vi "Auto State Machine.vi"   [LabVIEW 2013]
uses:
  typedefs/State Machine/singleUseSubstate.ctl
  typedefs/fg_typedef.ctl
  typedefs/State Machine/subStates.ctl
  typedefs/Vision/vision enable.ctl
  typedefs/DevRef Type.ctl
panel:
  # "A State Machine to Handle One or Two Ball Autonomous"
types:
  T1 = typedef "fg_typedef.ctl" = enum16{"Get", "Set"}
  T2 = typedef "singleUseSubstate.ctl" = enum16{"null", "wait", "shift high", "shift low", "extend shooter", "retract shooter", "latch", "unlatch", "end"}
  T3 = typedef "DevRef Type.ctl" = enum16{"Shooter Solenoid", "Latch Solenoid", "Right Up Sensor", "Right Down Sensor", "Hold Sensor", "2 Ball Switch", "Arm Encoder"}
  T4 = typedef "subStates.ctl" = enum16{"null", "wait", "driver control", "auto", "manual override", "hold position", "rotate", "pickup", "pass", "recover pass", "load", "goto shoot", "shoot high goal", "shoot low goal", "cancel arm", "cancel shooter", "end", "test"}
  T5 = typedef "vision enable.ctl" = enum16{"Enable", "Disable", "Stop"}
  T6 = typedef "WPI_EncoderDevRef.ctl" = cluster{"DevStatus":errorcluster, "EncoderIndex":T7, "CounterIndex":T8, "DistancePerCount":dbl, "Decoding Type":T9}
  T7 = typedef "FPGA_EncoderIdx.ctl" = enum8{"Enc 0", "Enc 1", "Enc 2", "Enc 3", "Invalid"}
  T8 = typedef "FPGA_CounterCtrSystemIndex.ctl" = enum8{"Ctr 0", "Ctr 1", "Ctr 2", "Ctr 3", "Ctr 4", "Ctr 5", "Ctr 6", "Ctr 7", "Invalid"}
  T9 = typedef "WPI_EncoderType.ctl" = enum16{"1x", "2x", "4x"}
  T10 = typedef "WPI_DigitalInputDevRef.ctl" = cluster{"DevStatus":errorcluster, "DIO Channel":T11, "Digital Module":T12}
  T11 = typedef "FPGA_DIOChannel.ctl" = enum8{"DIO 1", "DIO 2", "DIO 3", "DIO 4", "DIO 5", "DIO 6", "DIO 7", "DIO 8", "DIO 9", "DIO 10", "DIO 11", "DIO 12", "DIO 13", "DIO 14", "Invalid"}
  T12 = typedef "FPGA_TypedefDigitalModule.ctl" = enum16{"Digital Module 1", "Digital Module 2"}
  T13 = typedef "vision data.ctl" = cluster{"x":dbl, "y":dbl, "area":dbl, "width":dbl, "height":dbl, "Hot Goal Present?":bool, "distance":dbl}
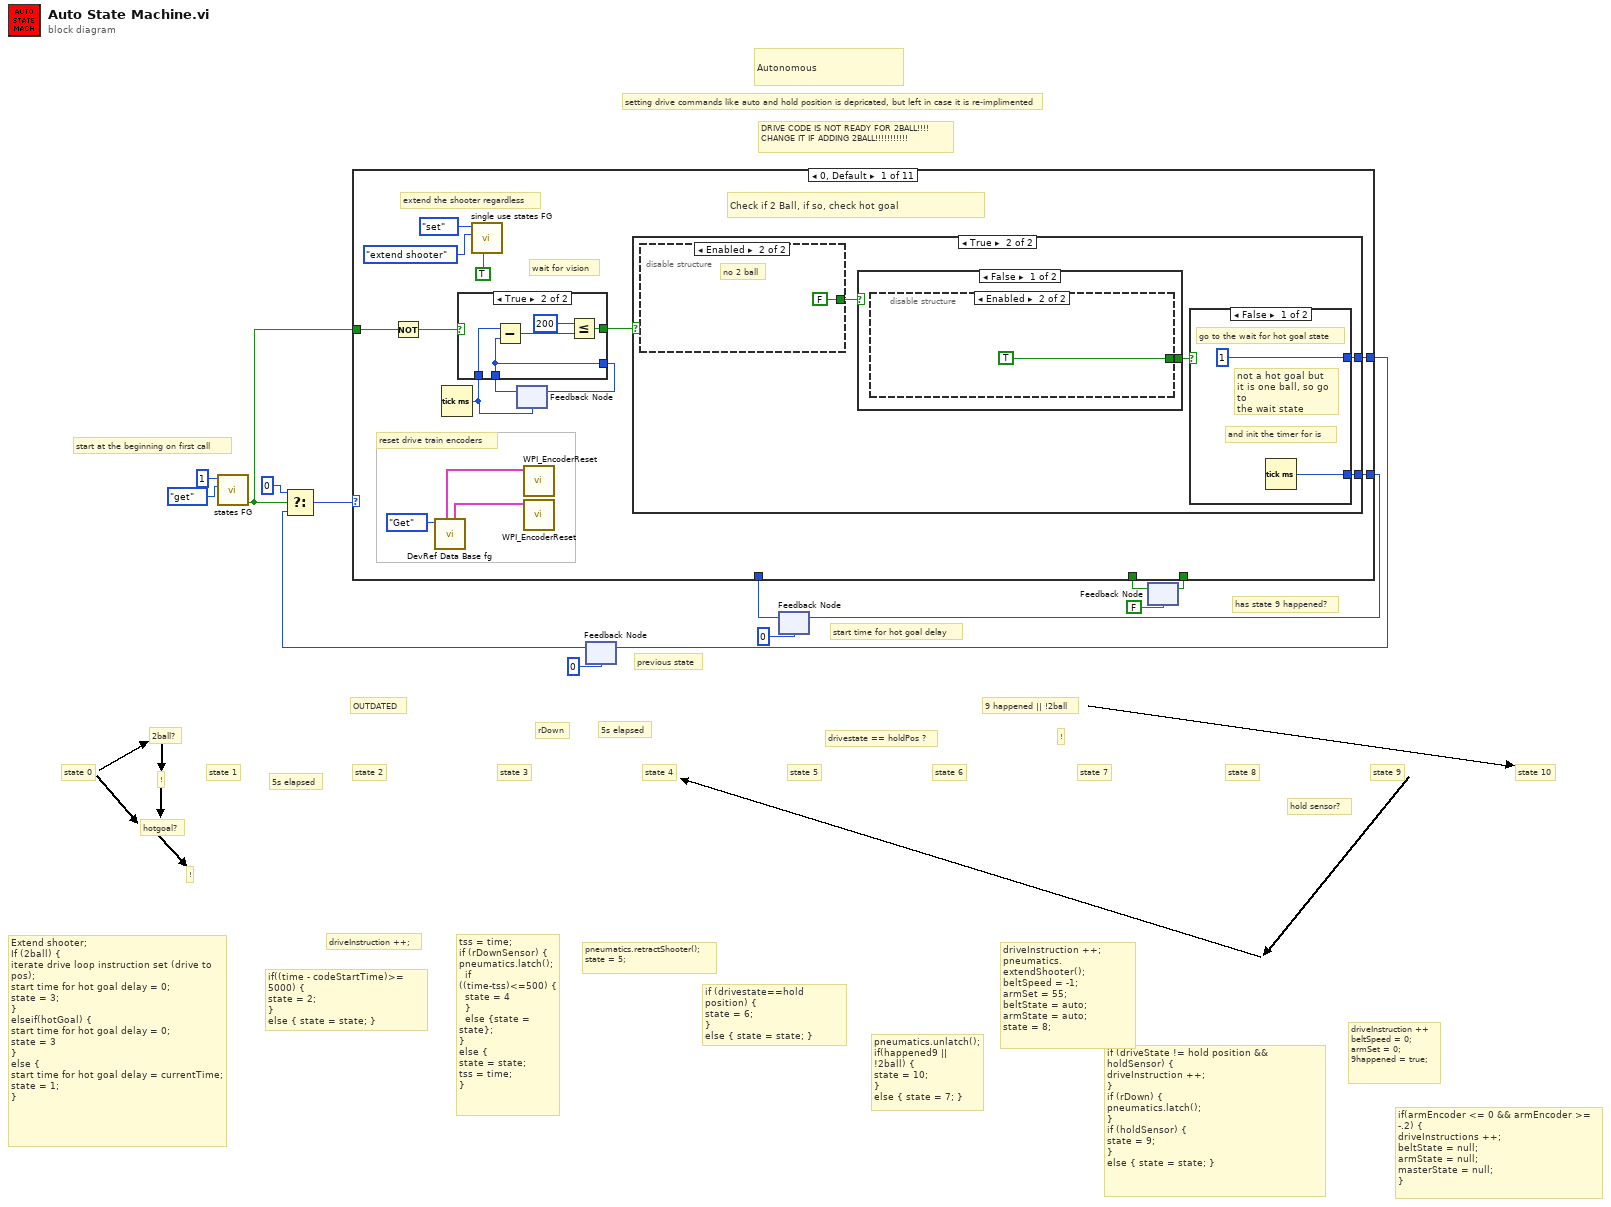
[diagram p0: block diagram]
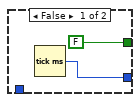
[diagram p2: hidden frame]
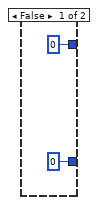
[diagram p3: hidden frame]
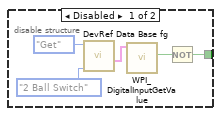
[diagram p4: hidden frame]
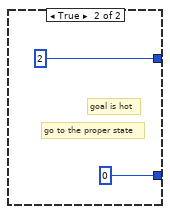
[diagram p5: hidden frame]
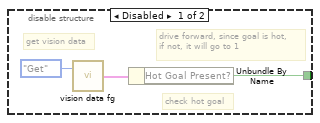
[diagram p6: hidden frame]
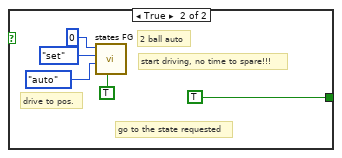
[diagram p7: hidden frame]
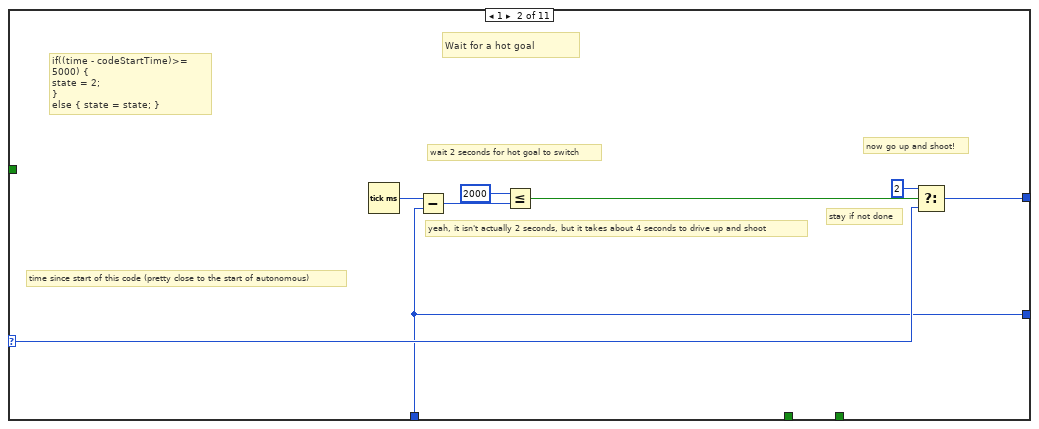
[diagram p8: hidden frame]
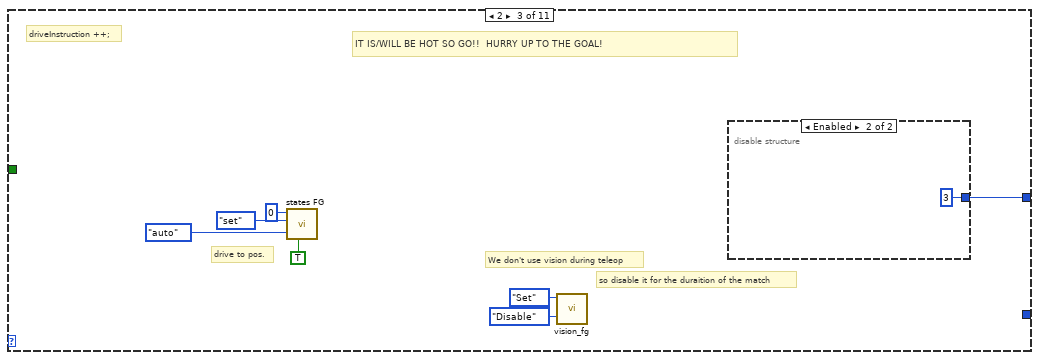
[diagram p9: hidden frame]
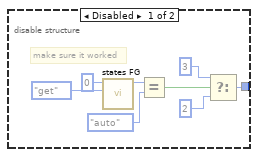
[diagram p10: hidden frame]
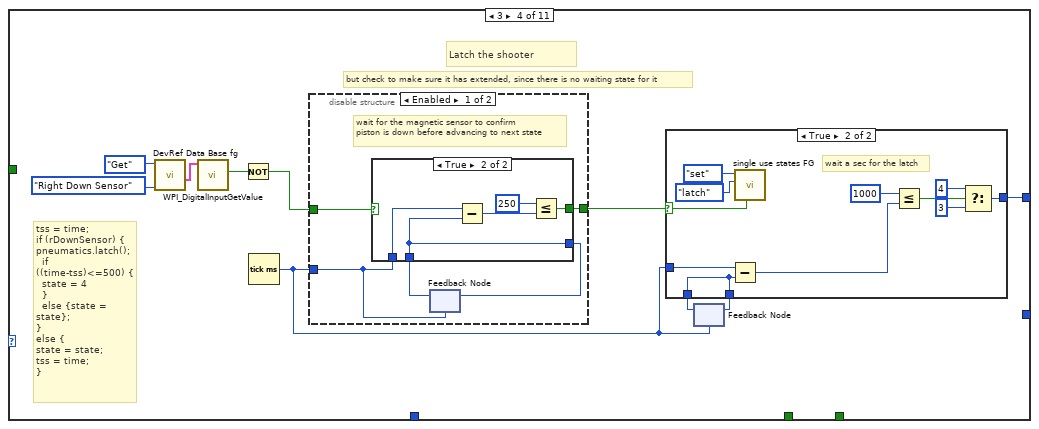
[diagram p11: hidden frame]
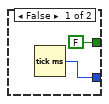
[diagram p12: hidden frame]
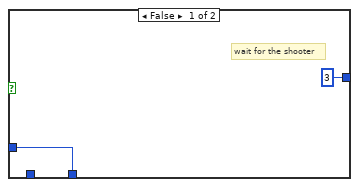
[diagram p14: hidden frame]
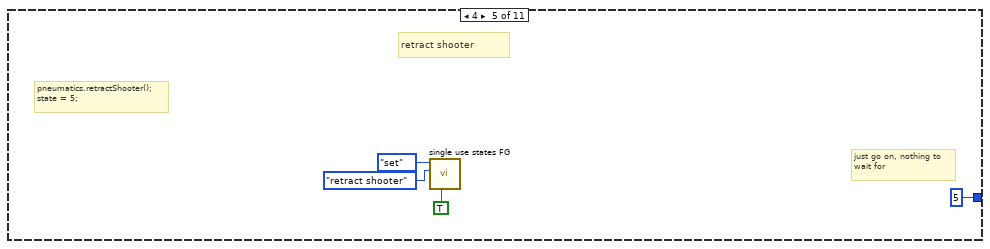
[diagram p15: hidden frame]
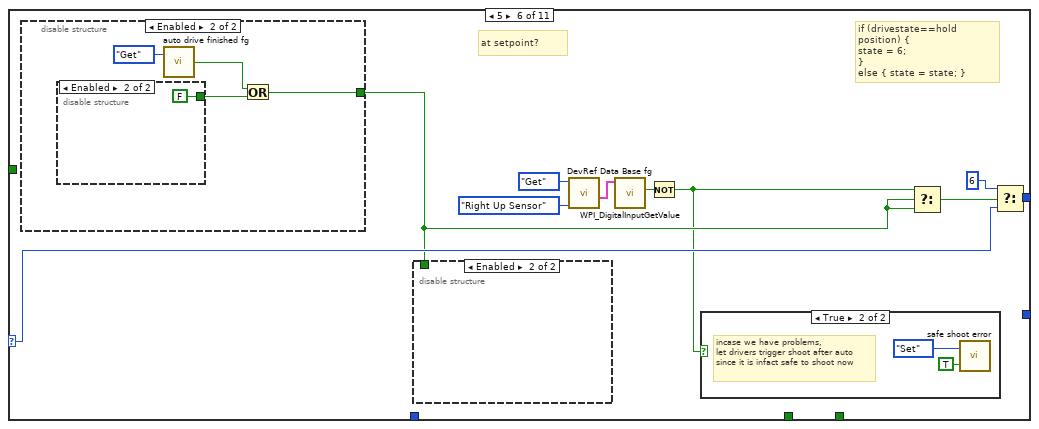
[diagram p16: hidden frame]
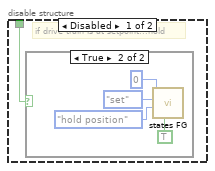
[diagram p17: hidden frame]
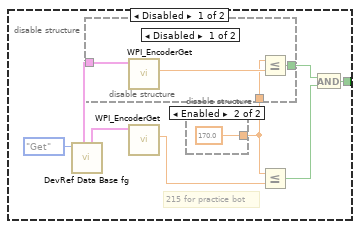
[diagram p19: hidden frame]
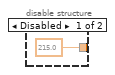
[diagram p20: hidden frame]
diagram:
  # "OUTDATED"
  # "DRIVE CODE IS NOT READY FOR 2BALL!!!!\nCHANGE IT IF ADDING 2BALL!!!!!!!!!!!"
  # "setting drive commands like auto and hold position is depricated, but left in case it is re-implimented"
  # "if(armEncoder <= 0 && armEncoder >= -.2) {\ndriveInstructions ++;\nbeltState = null;\narmState = null;\nmasterState = null;\n}"
  # "driveInstruction ++\nbeltSpeed = 0;\narmSet = 0;\n9happened = true;"
  # "if (driveState != hold position && holdSensor) {\ndriveInstruction ++;\n}\nif (rDown) {\npneumatics.latch();\n}\nif (holdSensor) {\nstate = 9;\n}\nelse { state = state; }"
  # "driveInstruction ++;\npneumatics.extendShooter();\nbeltSpeed = -1;\narmSet = 55;\nbeltState = auto;\narmState = auto;\nstate = 8;"
  # "pneumatics.unlatch();\nif(happened9 || !2ball) {\nstate = 10;\n}\nelse { state = 7; }"
  # "if (drivestate==hold position) {\nstate = 6;\n}\nelse { state = state; }"
  # "pneumatics.retractShooter();\nstate = 5;"
  # "tss = time;\nif (rDownSensor) {\npneumatics.latch();\n  if ((time-tss)<=500) {\n  state = 4\n  }\n  else {state = state};\n}\nelse {\nstate = state;\ntss = time;\n}"
  # "driveInstruction ++;"
  # "if((time - codeStartTime)>= 5000) {\nstate = 2;\n}\nelse { state = state; }"
  # "Extend shooter;\nIf (2ball) {\niterate drive loop instruction set (drive to pos);\nstart time for hot goal delay = 0;\nstate = 3;\n}\nelseif(hotGoal) {\nstart time for hot goal delay = 0;\nstate = 3\n}\nelse {\nstart time for hot goal delay = currentTime;\nstate = 1;\n}"
  # "hold sensor?"
  # "!"
  # "9 happened || !2ball"
  # "drivestate == holdPos ?"
  # "5s elapsed"
  # "rDown"
  # "5s elapsed"
  # "!"
  # "hotgoal?"
  # "!"
  # "state 10"
  # "2ball?"
  # "state 9"
  # "state 8"
  # "state 7"
  # "state 6"
  # "state 5"
  # "state 4"
  # "state 3"
  # "state 2"
  # "state 1"
  # "state 0"
  # "has state 9 happened?"
  # "start time for hot goal delay"
  # "previous state"
  # "start at the beginning on first call"
  # "Autonomous"
  n1 = call "states FG.vi"("menu (get)"=enum16{"set", "get"}."get", "Loop ID"=1) -> ("first call?"=w1:bool)  [unwired: 6 in, 3 out]
  n2 = feedback #1(u8 0) -> (w10:u8)
  n3 = Select(t=u8 0, s=w1, f=w10) -> (s? t:f=w12:u8)
  n4 = feedback #2(u32 0 ("millisecond timer value")) -> (w5:u32)
  n5 = feedback #3(FALSE) -> (w3:bool)
  n6 = case shown="0, Default" w12 {
    selector: w12 -> [_ w63 _ _ _ w135 _ _ w233 _ w269]
    tunnel: [w28 w64 w72 w91 u8 5 ("t") w133 w175 u8 8 ("t") w232 u8 4 ("t") w269] -> w8
    tunnel: [w27 w62 _ _ _ _ _ _ _ _ _] -> w7
    tunnel: w5 -> [_ w62 _ _ _ _ _ _ _ _ _]
    tunnel: [_ _ _ _ _ _ _ _ _ TRUE _] -> w4
    tunnel: w3 -> [_ _ _ _ _ _ w171 _ _ _ _]
    tunnel: w1 -> [w17 _ _ _ _ _ _ _ _ _ _]
    frame 0, Default {
      # "reset drive train encoders"
      # "wait for vision"
      # "extend the shooter regardless"
      # "Check if 2 Ball, if so, check hot goal"
      n7 = Not(x=w17) -> (.not. x?=w16:bool)
      n8 = call "DevRef Data Base fg.vi"("Menu"=fg_typedef."Get") -> ("right drive encoder"=w21:T6, "left drive encoder"=w22:T6)  [unwired: 3 in, 4 out]
      n9 = Tick Count (ms)() -> (millisecond timer value=w20:u32)
      n10 = call "single use states FG.vi"("exit in"=TRUE, "substate"=singleUseSubstate."extend shooter", "menu (get)"=enum16{"set", "get"}."set") -> ()  [unwired: 5 in, 4 out]
      n11 = feedback #4(w20) -> (w18:u32)
      n12 = case shown="True" w16 {
        tunnel: w20 -> [_ w33]
        tunnel: [w30 w31] -> w19
        tunnel: w18 -> [_ w31]
        tunnel: [FALSE w32] -> w15
        frame False {
          n13 = Tick Count (ms)() -> (millisecond timer value=w30:u32)
        }
        frame True {
          n14 = Subtract(x=w33, y=w31) -> (x-y=w35:u32)
          n15 = Less Or Equal?(x=u32 200, y=w35) -> (x <= y?=w32:bool)
        }
      }
      n16 = feedback-in #4(w19) -> ()
      n17 = call <vilib>:"WPI_EncoderReset.vi"("EncoderDevRef"=w22) -> ()  [unwired: 9 in, 2 out]
      n18 = call <vilib>:"WPI_EncoderReset.vi"("EncoderDevRef"=w21) -> ()  [unwired: 9 in, 2 out]
      n19 = case shown="True" w15 {
        tunnel: [u8 0 ("f") w40] -> w28
        tunnel: [u32 0 ("millisecond timer value") w39] -> w27
        frame False {
        }
        frame True {
          n20 = disable-structure shown="Enabled" {
            disable-tunnel: [w44 FALSE] -> w38
            frame Disabled {
              n21 = call "DevRef Data Base fg.vi"("DevRef to Get"=DevRef_Type."2 Ball Switch", "Menu"=fg_typedef."Get") -> ("Selected Sensor"=w46:T10)  [unwired: 2 in, 5 out]
              n22 = call <vilib>:"WPI_DigitalInputGetValue.vi"("DigitalInputDevRef"=w46) -> ("Value"=w45:bool)  [unwired: 8 in, 2 out]
              n23 = Not(x=w45) -> (.not. x?=w44:bool)
            }
            frame Enabled {
              # "no 2 ball"
            }
          }
          n24 = case shown="False" w38 {
            tunnel: [w52 TRUE ("Hot Goal Present?")] -> w41
            frame False {
              n25 = disable-structure shown="Enabled" {
                disable-tunnel: [w53 TRUE ("Hot Goal Present?")] -> w52
                frame Disabled {
                  # "drive forward, since goal is hot,\nif not, it will go to 1"
                  # "check hot goal"
                  # "get vision data"
                  n26 = call "vision data fg.vi"("Menu"=fg_typedef."Get") -> ("Output"=w54:T13)  [unwired: 1 in]
                  n27 = Unbundle By Name(w54) -> ("Hot Goal Present?"=w53:bool)
                }
                frame Enabled {
                }
              }
            }
            frame True {
              # "go to the state requested"
              # "drive to pos."
              # "start driving, no time to spare!!!"
              # "2 ball auto"
              n28 = call "states FG.vi"("exit in"=TRUE, "subState in"=subStates."auto", "menu (get)"=enum16{"set", "get"}."set", "Loop ID"=0) -> ()  [unwired: 4 in, 4 out]
            }
          }
          n29 = case shown="False" w41 {
            tunnel: [u8 1 ("f") u8 2] -> w40
            tunnel: [w49 u32 0 ("millisecond timer value")] -> w39
            frame False {
              # "go to the wait for hot goal state"
              # "and init the timer for is"
              # "not a hot goal but\nit is one ball, so go to\nthe wait state"
              n30 = Tick Count (ms)() -> (millisecond timer value=w49:u32)
            }
            frame True {
              # "go to the proper state"
              # "goal is hot"
            }
          }
        }
      }
    }
    frame 1 {
      # "yeah, it isn't actually 2 seconds, but it takes about 4 seconds to drive up and shoot"
      # "if((time - codeStartTime)>= 5000) {\nstate = 2;\n}\nelse { state = state; }"
      # "now go up and shoot!"
      # "stay if not done"
      # "time since start of this code (pretty close to the start of autonomous)"
      # "wait 2 seconds for hot goal to switch"
      # "Wait for a hot goal"
      n31 = Tick Count (ms)() -> (millisecond timer value=w67:u32)
      n32 = Subtract(x=w67, y=w62) -> (x-y=w69:u32)
      n33 = Less Or Equal?(x=u32 2000, y=w69) -> (x <= y?=w66:bool)
      n34 = Select(t=u8 2, s=w66, f=w63) -> (s? t:f=w64:u8)
    }
    frame 2 {
      # "so disable it for the duraition of the match"
      # "We don't use vision during teleop"
      # "driveInstruction ++;"
      # "drive to pos."
      # "IT IS/WILL BE HOT SO GO!!  HURRY UP TO THE GOAL!"
      n35 = call "states FG.vi"("exit in"=TRUE, "subState in"=subStates."auto", "menu (get)"=enum16{"set", "get"}."set", "Loop ID"=0) -> ()  [unwired: 4 in, 4 out]
      n36 = call "vision_fg.vi"("Action"=vision_enable."Disable", "Menu"=fg_typedef."Set" ("Enum")) -> ()  [unwired: 1 in, 2 out]
      n37 = disable-structure shown="Enabled" {
        disable-tunnel: [w77 u8 3 ("t")] -> w72
        frame Disabled {
          # "make sure it worked"
          n38 = call "states FG.vi"("menu (get)"=enum16{"set", "get"}."get", "Loop ID"=0) -> ("subState out"=w82:T4)  [unwired: 6 in, 3 out]
          n39 = Equal?(x=w82, y=subStates."auto" ("subState in")) -> (x = y?=w80:bool)
          n40 = Select(t=u8 3, s=w80, f=u8 2 ("t")) -> (s? t:f=w77:u8)
        }
        frame Enabled {
        }
      }
    }
    frame 3 {
      # "tss = time;\nif (rDownSensor) {\npneumatics.latch();\n  if ((time-tss)<=500) {\n  state = 4\n  }\n  else {state = state};\n}\nelse {\nstate = state;\ntss = time;\n}"
      # "but check to make sure it has extended, since there is no waiting state for it"
      # "Latch the shooter"
      n41 = call "DevRef Data Base fg.vi"("DevRef to Get"=DevRef_Type."Right Down Sensor", "Menu"=fg_typedef."Get") -> ("Selected Sensor"=w95:T10)  [unwired: 2 in, 5 out]
      n42 = call <vilib>:"WPI_DigitalInputGetValue.vi"("DigitalInputDevRef"=w95) -> ("Value"=w94:bool)  [unwired: 8 in, 2 out]
      n43 = Not(x=w94) -> (.not. x?=w88:bool)
      n44 = Tick Count (ms)() -> (millisecond timer value=w87:u32)
      n45 = disable-structure shown="Enabled" {
        disable-tunnel: w88 -> [w100 w108]
        disable-tunnel: [w97 w108] -> w86
        disable-tunnel: w87 -> [w96 _]
        frame Enabled {
          # "wait for the magnetic sensor to confirm \npiston is down before advancing to next state"
          n46 = feedback #5(w96) -> (w98:u32)
          n47 = case shown="True" w100 {
            tunnel: w96 -> [_ w105]
            tunnel: [w102 w103] -> w99
            tunnel: w98 -> [_ w103]
            tunnel: [FALSE w104] -> w97
            frame False {
              n48 = Tick Count (ms)() -> (millisecond timer value=w102:u32)
            }
            frame True {
              n49 = Subtract(x=w105, y=w103) -> (x-y=w107:u32)
              n50 = Less Or Equal?(x=u32 250, y=w107) -> (x <= y?=w104:bool)
            }
          }
          n51 = feedback-in #5(w99) -> ()
        }
        frame Disabled {
        }
      }
      n52 = feedback #6(w87) -> (w92:u32)
      n53 = case shown="True" w86 {
        selector: w86 -> [_ w117]
        tunnel: [w109 w119] -> w93
        tunnel: w92 -> [_ w119]
        tunnel: w87 -> [w109 w118]
        tunnel: [u8 3 ("f") w112] -> w91
        frame False {
          # "wait for the shooter"
        }
        frame True {
          # "wait a sec for the latch"
          n54 = Subtract(x=w118, y=w119) -> (x-y=w114:u32)
          n55 = call "single use states FG.vi"("exit in"=w117, "substate"=singleUseSubstate."latch", "menu (get)"=enum16{"set", "get"}."set") -> ()  [unwired: 5 in, 4 out]
          n56 = Less Or Equal?(x=u32 1000, y=w114) -> (x <= y?=w111:bool)
          n57 = Select(t=u8 4, s=w111, f=u8 3) -> (s? t:f=w112:u8)
        }
      }
      n58 = feedback-in #6(w93) -> ()
    }
    frame 4 {
      # "pneumatics.retractShooter();\nstate = 5;"
      # "just go on, nothing to\nwait for"
      # "retract shooter"
      n59 = call "single use states FG.vi"("exit in"=TRUE, "substate"=singleUseSubstate."retract shooter", "menu (get)"=enum16{"set", "get"}."set") -> ()  [unwired: 5 in, 4 out]
    }
    frame 5 {
      # "if (drivestate==hold position) {\nstate = 6;\n}\nelse { state = state; }"
      # "at setpoint?"
      n60 = disable-structure shown="Enabled" {
        disable-tunnel: [w141 w156] -> w127
        frame Disabled {
          # "215 for practice bot"
          n61 = call "DevRef Data Base fg.vi"("Menu"=fg_typedef."Get") -> ("right drive encoder"=w147:T6, "left drive encoder"=w146:T6)  [unwired: 3 in, 4 out]
          n62 = call <vilib>:"WPI_EncoderGet.vi"("EncoderDevRef"=w147) -> ("Distance"=w145:dbl)  [unwired: 5 in, 5 out]
          n63 = disable-structure shown="Enabled" {
            disable-tunnel: [215.0 ("x") 170.0 ("x")] -> w142
            frame Disabled {
            }
            frame Enabled {
            }
          }
          n64 = disable-structure shown="Disabled" {
            disable-tunnel: w146 -> [w154 _]
            disable-tunnel: [w152 TRUE] -> w144
            disable-tunnel: w142 -> [w151 _]
            frame Disabled {
              n65 = call <vilib>:"WPI_EncoderGet.vi"("EncoderDevRef"=w154) -> ("Distance"=w153:dbl)  [unwired: 5 in, 5 out]
              n66 = Less Or Equal?(x=w151, y=w153) -> (x <= y?=w152:bool)
            }
            frame Enabled {
            }
          }
          n67 = Less Or Equal?(x=w142, y=w145) -> (x <= y?=w143:bool)
          n68 = And(x=w144, y=w143) -> (x .and. y?=w141:bool)
        }
        frame Enabled {
          n69 = disable-structure shown="Enabled" {
            disable-tunnel: [w160 FALSE] -> w157
            frame Disabled {
              # "check if drive is in hold"
              n70 = call "states FG.vi"("menu (get)"=enum16{"set", "get"}."get", "Loop ID"=0) -> ("subState out"=w162:T4)  [unwired: 6 in, 3 out]
              n71 = Equal?(x=w162, y=subStates."hold position" ("subState in")) -> (x = y?=w160:bool)
            }
            frame Enabled {
            }
          }
          n72 = call "auto drive finished fg.vi"("Menu"=fg_typedef."Get") -> ("Done"=w158:bool)  [unwired: 1 in]
          n73 = Or(x=w158, y=w157) -> (x .or. y?=w156:bool)
        }
      }
      n74 = disable-structure shown="Enabled" {
        disable-tunnel: w127 -> [w136 _]
        frame Disabled {
          # "if drive train is at setpoint...hold"
          n75 = case shown="True" w136 {
            frame False {
            }
            frame True {
              n76 = call "states FG.vi"("exit in"=TRUE, "subState in"=subStates."hold position" ("y"), "menu (get)"=enum16{"set", "get"}."set", "Loop ID"=0) -> ()  [unwired: 4 in, 4 out]
            }
          }
        }
        frame Enabled {
        }
      }
      n77 = call "DevRef Data Base fg.vi"("DevRef to Get"=DevRef_Type."Right Up Sensor", "Menu"=fg_typedef."Get") -> ("Selected Sensor"=w132:T10)  [unwired: 2 in, 5 out]
      n78 = call <vilib>:"WPI_DigitalInputGetValue.vi"("DigitalInputDevRef"=w132) -> ("Value"=w131:bool)  [unwired: 8 in, 2 out]
      n79 = Not(x=w131) -> (.not. x?=w126:bool)
      n80 = case shown="True" w126 {
        frame False {
        }
        frame True {
          # "incase we have problems,\nlet drivers trigger shoot after auto\nsince it is infact safe to shoot now"
          n81 = call "safe shoot error.vi"("Can Shoot Safely?"=TRUE, "Menu"=fg_typedef."Set") -> ()  [unwired: 1 out]
        }
      }
      n82 = Select(t=w126, s=w127, f=w127) -> (s? t:f=w128:bool)
      n83 = Select(t=u8 6, s=w128, f=w135) -> (s? t:f=w133:u8)
    }
    frame 6 {
      w169 = FALSE ("Can Shoot Safely?")
      w168 = fg_typedef."Set" ("Menu")
      # "no 2 ball auto ever (as of now)"
      # "unlatch shooter"
      # "SHOOT!!!"
      n84 = call "safe shoot error.vi"("Can Shoot Safely?"=w169, "Menu"=w168) -> ()  [unwired: 1 out]
      n85 = call "auto drive finished fg.vi"("Done?"=w169, "Menu"=w168) -> ()  [unwired: 1 out]
      n86 = call "single use states FG.vi"("exit in"=TRUE, "substate"=singleUseSubstate."unlatch", "menu (get)"=enum16{"set", "get"}."set") -> ()  [unwired: 5 in, 4 out]
      n87 = disable-structure shown="Enabled" {
        disable-tunnel: [w178 TRUE ("Value")] -> w170
        frame Disabled {
          n88 = call "DevRef Data Base fg.vi"("DevRef to Get"=DevRef_Type."2 Ball Switch", "Menu"=fg_typedef."Get") -> ("Selected Sensor"=w179:T10)  [unwired: 2 in, 5 out]
          n89 = call <vilib>:"WPI_DigitalInputGetValue.vi"("DigitalInputDevRef"=w179) -> ("Value"=w178:bool)  [unwired: 8 in, 2 out]
        }
        frame Enabled {
        }
      }
      n90 = disable-structure shown="Enabled" {
        disable-tunnel: [w187 w190] -> w175
        disable-tunnel: w171 -> [w185 w194]
        disable-tunnel: w170 -> [w184 w189]
        frame Disabled {
          # "pneumatics.unlatch();\nif(happened9) {\nstate = 10;\n}\nelseif(2ball) {\nstate = 7\n}\nelse {\nstate = 10\n}"
          # "if 2 ball was done,\ngo on to 7"
          # "prepare for a 2nd ball"
          # "null if done"
          n91 = Not(x=w184) -> (.not. x?=w181:bool)
          n92 = Select(t=FALSE, s=w185, f=w181) -> (s? t:f=w182:bool)
          n93 = Select(t=u8 7, s=w182, f=u8 10 ("t")) -> (s? t:f=w187:u8)
        }
        frame Enabled {
          # "pneumatics.unlatch();\nif(happened9 || !2ball) {\nstate = 10;\n}\nelse { state = 7; }"
          n94 = disable-structure shown="Enabled" {
            disable-tunnel: w194 -> [w197 _]
            disable-tunnel: [w196 w198] -> w193
            disable-tunnel: w189 -> [w195 w198]
            frame Disabled {
              n95 = Or(x=w195, y=w197) -> (x .or. y?=w196:bool)
            }
            frame Enabled {
            }
          }
          n96 = Select(t=u8 10, s=w193, f=u8 7 ("t")) -> (s? t:f=w190:u8)
        }
      }
    }
    frame 7 {
      # "drive back now"
      # "prepare for a ball"
      # "arm to up position"
      # "enable belts and arm"
      # "driveInstruction ++;\npneumatics.extendShooter();\nbeltSpeed = -1;\narmSet = 55;\nbeltState = auto;\narmState = auto;\nstate = 8;"
      # "belts in"
      # "run load commands, drive backwards"
      n97 = call "states FG.vi"("exit in"=TRUE, "menu (get)"=enum16{"set", "get"}."set", "Loop ID"=0) -> ()  [unwired: 5 in, 4 out]
      n98 = call "single use states FG.vi"("exit in"=TRUE, "substate"=singleUseSubstate."extend shooter", "menu (get)"=enum16{"set", "get"}."set") -> ()  [unwired: 5 in, 4 out]
      n99 = call "Arm Setpoint FG.vi"("Setpoint In"=55.0, "Menu"=fg_typedef."Set") -> ()  [unwired: 1 out]
      n100 = call "Belt Speed FG.vi"("Speed In"=-1.0, "Menu"=fg_typedef."Set") -> ()  [unwired: 1 out]
      n101 = call "states FG.vi"("exit in"=TRUE, "subState in"=subStates."auto", "menu (get)"=enum16{"set", "get"}."set", "Loop ID"=2) -> ()  [unwired: 4 in, 4 out]
      n102 = call "states FG.vi"("exit in"=TRUE, "subState in"=subStates."auto", "menu (get)"=enum16{"set", "get"}."set", "Loop ID"=3) -> ()  [unwired: 4 in, 4 out]
    }
    frame 8 {
      # "if (driveState != hold position && holdSensor) {\ndriveInstruction ++;\n}\nif (rDown) {\npneumatics.latch();\n}\nif (holdSensor) {\nstate = 9;\n}\nelse { state = state; }"
      # "latch if extended"
      # "have ball?"
      n103 = disable-structure shown="Enabled" {
        disable-tunnel: [w235 w240] -> w227
        frame Disabled {
          n104 = call "states FG.vi"("menu (get)"=enum16{"set", "get"}."get", "Loop ID"=0) -> ("subState out"=w237:T4)  [unwired: 6 in, 3 out]
          n105 = Not Equal?(x=w237, y=subStates."hold position") -> (x != y?=w235:bool)
        }
        frame Enabled {
          # "if it is close enough..."
          n106 = call "DevRef Data Base fg.vi"("Menu"=fg_typedef."Get") -> ("right drive encoder"=w242:T6, "left drive encoder"=w241:T6)  [unwired: 3 in, 4 out]
          n107 = call <vilib>:"WPI_EncoderGet.vi"("EncoderDevRef"=w241) -> ("Distance"=w249:dbl)  [unwired: 5 in, 5 out]
          n108 = call <vilib>:"WPI_EncoderGet.vi"("EncoderDevRef"=w242) -> ("Distance"=w248:dbl)  [unwired: 5 in, 5 out]
          n109 = Add(x=w249, y=w248) -> (x+y=w247:dbl)
          n110 = Divide(x=w247, y=2.0) -> (x/y=w245:dbl)
          n111 = Greater Or Equal?(x=10.0, y=w245) -> (x >= y?=w240:bool)
        }
      }
      n112 = call "DevRef Data Base fg.vi"("DevRef to Get"=DevRef_Type."Hold Sensor", "Menu"=fg_typedef."Get") -> ("Selected Sensor"=w231:T10)  [unwired: 2 in, 5 out]
      n113 = call "DevRef Data Base fg.vi"("DevRef to Get"=DevRef_Type."Right Down Sensor", "Menu"=fg_typedef."Get") -> ("Selected Sensor"=w226:T10)  [unwired: 2 in, 5 out]
      n114 = call <vilib>:"WPI_DigitalInputGetValue.vi"("DigitalInputDevRef"=w231) -> ("Value"=w230:bool)  [unwired: 8 in, 2 out]
      n115 = call <vilib>:"WPI_DigitalInputGetValue.vi"("DigitalInputDevRef"=w226) -> ("Value"=w225:bool)  [unwired: 8 in, 2 out]
      n116 = Not(x=w225) -> (.not. x?=w224:bool)
      n117 = Not(x=w230) -> (.not. x?=w228:bool)
      n118 = case shown="True" w224 {
        tunnel: [FALSE w251] -> w222
        frame False {
          # "wait.."
        }
        frame True {
          w251 = TRUE
          n119 = call "single use states FG.vi"("exit in"=w251, "substate"=singleUseSubstate."latch", "menu (get)"=enum16{"set", "get"}."set") -> ()  [unwired: 5 in, 4 out]
        }
      }
      n120 = And(x=w227, y=w228) -> (x .and. y?=w229:bool)
      n121 = case shown="True" w229 {
        frame False {
        }
        frame True {
          # "stop drive if it is not already"
          n122 = call "states FG.vi"("exit in"=TRUE, "subState in"=subStates."hold position", "menu (get)"=enum16{"set", "get"}."set", "Loop ID"=0) -> ()  [unwired: 4 in, 4 out]
        }
      }
      n123 = And(x=w228, y=w222) -> (x .and. y?=w223:bool)
      n124 = Select(t=u8 9, s=w223, f=w233) -> (s? t:f=w232:u8)
    }
    frame 9 {
      # "driveInstruction ++\nbeltSpeed = 0;\narmSet = 0;\n9happened = true;"
      # "arm down"
      # "belts off"
      # "sends drive into auto state (due to autonomous code setup)"
      # "drive to pos."
      # "drive forward, arm down, belts off"
      n125 = call "states FG.vi"("exit in"=TRUE, "subState in"=subStates."auto", "menu (get)"=enum16{"set", "get"}."set", "Loop ID"=0) -> ()  [unwired: 4 in, 4 out]
      n126 = call "Arm Setpoint FG.vi"("Setpoint In"=0.0, "Menu"=fg_typedef."Set") -> ()  [unwired: 1 out]
      n127 = call "Belt Speed FG.vi"("Speed In"=0.0, "Menu"=fg_typedef."Set") -> ()  [unwired: 1 out]
    }
    frame 10 {
      # "if(armEncoder <= 0 && armEncoder >= -.2) {\ndriveInstructions ++;\nbeltState = null;\narmState = null;\nmasterState = null;\n}"
      # "null all the things"
      n128 = disable-structure shown="Enabled" {
        disable-tunnel: [w272 TRUE] -> w268
        frame Disabled {
          n129 = call "DevRef Data Base fg.vi"("DevRef to Get"=DevRef_Type."2 Ball Switch", "Menu"=fg_typedef."Get") -> ("Selected Encoder"=w276:T6)  [unwired: 2 in, 5 out]
          n130 = call <vilib>:"WPI_EncoderGet.vi"("EncoderDevRef"=w276) -> ("Distance"=w275:dbl)  [unwired: 5 in, 5 out]
          n131 = In Range and Coerce(upper limit=1.0, x=w275, lower limit=-0.4) -> (In Range?=w272:bool)  [unwired: 1 out]
        }
        frame Enabled {
        }
      }
      n132 = case shown="True" w268 {
        frame False {
        }
        frame True {
          # "null things"
          n133 = call "states FG.vi"("exit in"=TRUE, "subState in"=subStates."null", "menu (get)"=enum16{"set", "get"}."set", "Loop ID"=0) -> ()  [unwired: 4 in, 4 out]
          n134 = call "states FG.vi"("exit in"=TRUE, "subState in"=subStates."null", "menu (get)"=enum16{"set", "get"}."set", "Loop ID"=1) -> ()  [unwired: 4 in, 4 out]
          n135 = call "states FG.vi"("exit in"=TRUE, "subState in"=subStates."null", "menu (get)"=enum16{"set", "get"}."set", "Loop ID"=2) -> ()  [unwired: 4 in, 4 out]
          n136 = call "states FG.vi"("exit in"=TRUE, "subState in"=subStates."null", "menu (get)"=enum16{"set", "get"}."set", "Loop ID"=3) -> ()  [unwired: 4 in, 4 out]
        }
      }
    }
  }
  n137 = feedback-in #1(w8) -> ()
  n138 = feedback-in #2(w7) -> ()
  n139 = feedback-in #3(w4) -> ()
